vi "Array_2D_Reduce_Sum_Dim=1.vi"(11 "x":sgl[][](array[numeric])) -> (3 "x out":sgl[](array[numeric]))   [LabVIEW 2020]
uses:
  <vilib>/addons/Multicore Analysis and Sparse Matrix/BLAS/_blas/sgemv - General Matrix-Vector Product (SGL).vi
  <vilib>/addons/Multicore Analysis and Sparse Matrix/Linear Algebra/NI_MASM_BasicLinAlg.lvlib
  <vilib>/addons/Multicore Analysis and Sparse Matrix/Linear Algebra/_linalg/Transpose Matrix (SGL).vi
  <vilib>/addons/Multicore Analysis and Sparse Matrix/BLAS/NI_MASM_BLAS.lvlib
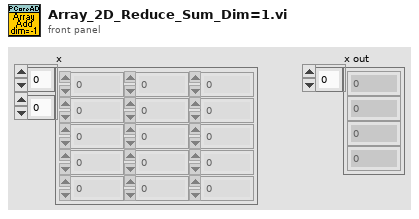
[diagram p1: front panel]
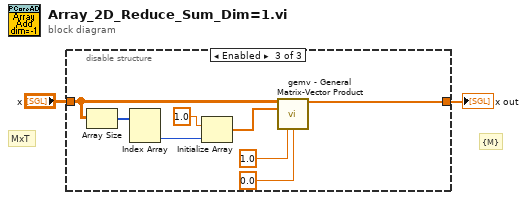
[diagram p0: block diagram]
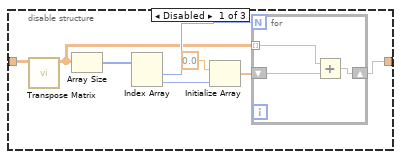
[diagram p2: hidden frame]
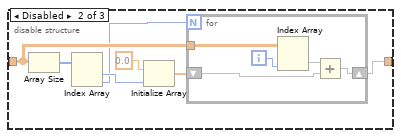
[diagram p3: hidden frame]
diagram:
  # "{M}"
  # "MxT"
  n1 = disable-structure shown="Enabled" {
    disable-tunnel: "x" -> [w10 w20 w31]
    disable-tunnel: [w9 w19 w27] -> w1
    frame Disabled {
      n2 = call-poly <vilib>:"Transpose Matrix.vi"("Input Matrix"=w10) -> ("Matrix Transpose"=w4:sgl[][])  [unwired: 9 in, 1 out]
      n3 = Array Size(array=w4) -> (size(s)=w8:i32[])
      n4 = Index Array(array=w8) -> (element #1=w6:i32, element #2=w3:i32)  [unwired: 2 in]
      n5 = Initialize Array(sgl 0.0 ("element"), w3) -> (w5:sgl[])
      n6 = for {
        N: w6 -> [_]
        tunnel: w4 -> [w13] mode=indexing
        shift-right: [w12] -> w9
        shift-left: w5 -> [w11]
        n7 = Add(x=w13, y=w11) -> (x+y=w12:sgl[])
      }
    }
    frame Disabled {
      n8 = Array Size(array=w20) -> (size(s)=w18:i32[])
      n9 = Index Array(array=w18) -> (element #1=w16:i32, element #2=w15:i32)  [unwired: 2 in]
      n10 = Initialize Array(sgl 0.0 ("element"), w16) -> (w14:sgl[])
      n11 = for {
        N: w15 -> [_]
        tunnel: w20 -> [w25]
        shift-right: [w23] -> w19
        shift-left: w14 -> [w22]
        i -> [w21]
        n12 = Index Array(array=w25, index (col)=w21) -> (element=w24:sgl[])  [unwired: 1 in]
        n13 = Add(x=w24, y=w22) -> (x+y=w23:sgl[])
      }
    }
    frame Enabled {
      n14 = Array Size(array=w31) -> (size(s)=w33:i32[])
      n15 = Index Array(array=w33) -> (element #2=w26:i32)  [unwired: 2 in, 1 out]
      n16 = Initialize Array(sgl 1.0 ("element"), w26) -> (w30:sgl[])
      n17 = call-poly <vilib>:"gemv - General Matrix-Vector Product.vi"("A"=w31, "x"=w30, "alpha"=sgl 1.0, "beta"=sgl 0.0) -> ("sgemv"=w27:sgl[])  [unwired: 10 in, 1 out]
    }
  }
  "x out" <- w1
